vi "Element Type.vi"(11 "BooleanIndicator in":refnum<class "BooleanIndicator.lvclass">) -> (2 "Element Type":string)   [LabVIEW 2020, in "VolatusGUIElements.lvlib" / "BooleanIndicator.lvclass"]
uses:
  BooleanIndicator.lvclass
  BooleanIndicator.lvclass/BooleanIndicator.ctl
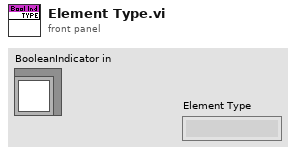
[diagram p1: front panel]
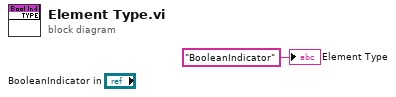
[diagram p0: block diagram]
diagram:
  "Element Type" <- "BooleanIndicator" ("Element Type")
